vi "例10.9  读取单幅图像.vi"() -> ()   [LabVIEW 2017]
panel:
  out "图像":T1(plugin-control)
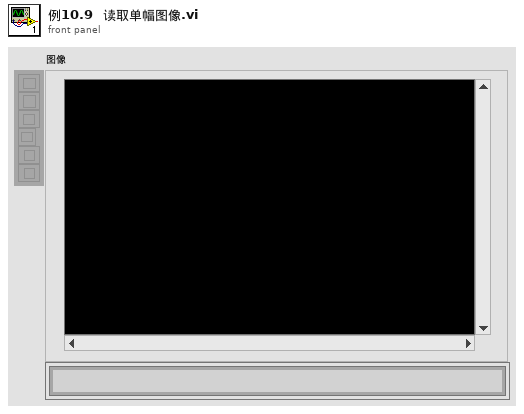
[diagram p1: front panel]
types:
  T1 = typedef "IMAQ Image.ctl" = refnum<image>
  T2 = typedef "Image Type" = u32
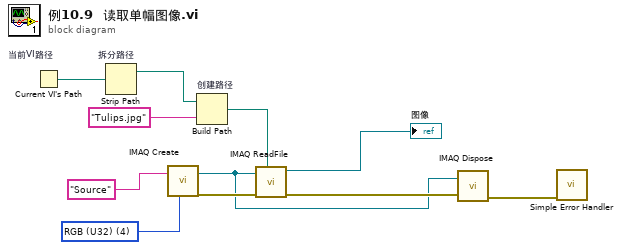
[diagram p0: block diagram]
diagram:
  w3 = T2 4 items=["Grayscale (U8)", "Grayscale (I16)", "Grayscale (SGL)", "Complex (CSG)", "RGB (U32)", "HSL (U32)", "RGB (U64)", "Grayscale (U16)"] ("Image Type")
  n1 = Current VI's Path "当前VI路径"() -> (path=w6:path)
  n2 = Strip Path "拆分路径"(path=w6) -> (stripped path=w5:path)  [unwired: 1 out]
  n3 = call "IMAQ Create"("Image Name"="Source", "Image Type"=w3) -> ("New Image"=w1:T1, "error out"=w10:errorcluster)  [unwired: 2 in, 1 out]
  n4 = Build Path "创建路径"(base path=w5, name or relative path="Tulips.jpg") -> (appended path=w4:path)
  n5 = call "IMAQ ReadFile"("File Path"=w4, "error in (no error)"=w10, "Image"=w1) -> ("error out"=w7:errorcluster, "Image Out"=→"图像":T1)  [unwired: 2 in, 5 out]
  n6 = call "IMAQ Dispose"("Image"=w1, "error in (no error)"=w7) -> ("error out"=w8:errorcluster)  [unwired: 1 in, 3 out]
  n7 = call <vilib>:"Simple Error Handler.vi"("error in (no error)"=w8) -> ()  [unwired: 1 in, 8 out]
